vi "Main.vi"(8 "error in (no error)":errorcluster, 11 "ModuleAdmin":refnum<class "ModuleAdmin.lvclass">) -> ()   [LabVIEW 2014, in "MyPluggableModule.lvlib"]
uses:
  MyPluggableModule.lvlib
  <userlib>/NIST/ModuleAdminLib/ModuleAdmin/ModuleAdmin.lvclass
  MyPlugins/MyPluginBaseClass/MyPluginsBase.lvclass
  PublicAPI/Arguments/Requests/clStopArgument.ctl
  <userlib>/NIST/ModuleAdminLib/ModuleAdmin/ModuleAdmin.lvclass/ModuleAdmin.ctl
  <userlib>/NIST/BaseClasses/BasePlugin_class/BasePlugin.lvclass/BasePlugin.ctl
  <vilib>/Utility/error.llb/DialogType.ctl
  <userlib>/NIST/ModuleAdminLib/ModuleAdmin/Accessors/Read ShowPanel_.vi
  <userlib>/NIST/ModuleAdminLib/ModuleAdmin/Accessors/Write ShowPanel_.vi
  <userlib>/NIST/BaseClasses/BasePlugin_class/Accessors/Write PluginIniFilePath.vi
  <userlib>/NIST/BaseClasses/BasePlugin_class/Accessors/Read PluginIniFilePath.vi
  <userlib>/NIST/ModuleAdminLib/ModuleAdmin/Accessors/Read CloneRegRef.vi
  <vilib>/Utility/error.llb/Error Cluster From Error Code.vi
  <vilib>/ErrorRing/Error Ring.xnode
  <userlib>/NIST/ModuleAdminLib/CloneRegistration/CloneRegistration.lvclass
  <userlib>/NIST/BaseClasses/Object_class/BaseObject.lvclass
  <userlib>/NIST/ModuleAdminLib/ModuleAdmin.lvlib
panel:
  out "error out":errorcluster
  # "This is the template for your cloneable module.\nYou should modifiy this to perform the functionality\nthat you want it to perform"
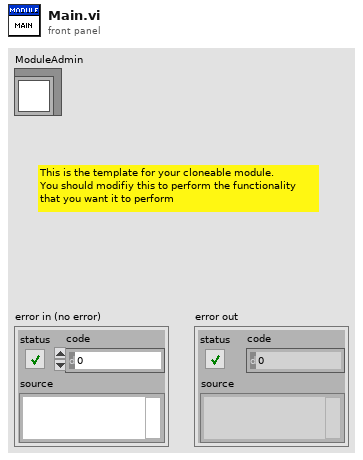
[diagram p1: front panel]
types:
  T1 = typedef "MyPluggableModule.lvlib/clRequestEvents.ctl" = cluster{"StopRequest":refnum<user-event>, "PathToINI":refnum<user-event>, " LoadPlugin":refnum<user-event>, "ShowPanel":refnum<user-event>, "PrefDlg":refnum<user-event>}
  T2 = typedef "MyPluggableModule.lvlib/clBroadcastEvents.ctl" = cluster{"DidInit":refnum<user-event>, "StatusUpdate":refnum<user-event>, "ErrorReport":refnum<user-event>, "DidStop":refnum<user-event>, "PathToINI":refnum<user-event>}
  T3 = typedef "MyPluggableModule.lvlib/clStopArgument.ctl" = cluster{"Exit via Stop Module Req?":bool, "Wait for Module to stop?":bool, "ModuleAdmin":refnum<class "ModuleAdmin.lvclass">}
  T4 = enum32{"Invalid", "Standard", "Closed", "Hidden", "Minimized", "Maximized"}
  T5 = typedef "DialogType.ctl" = u16
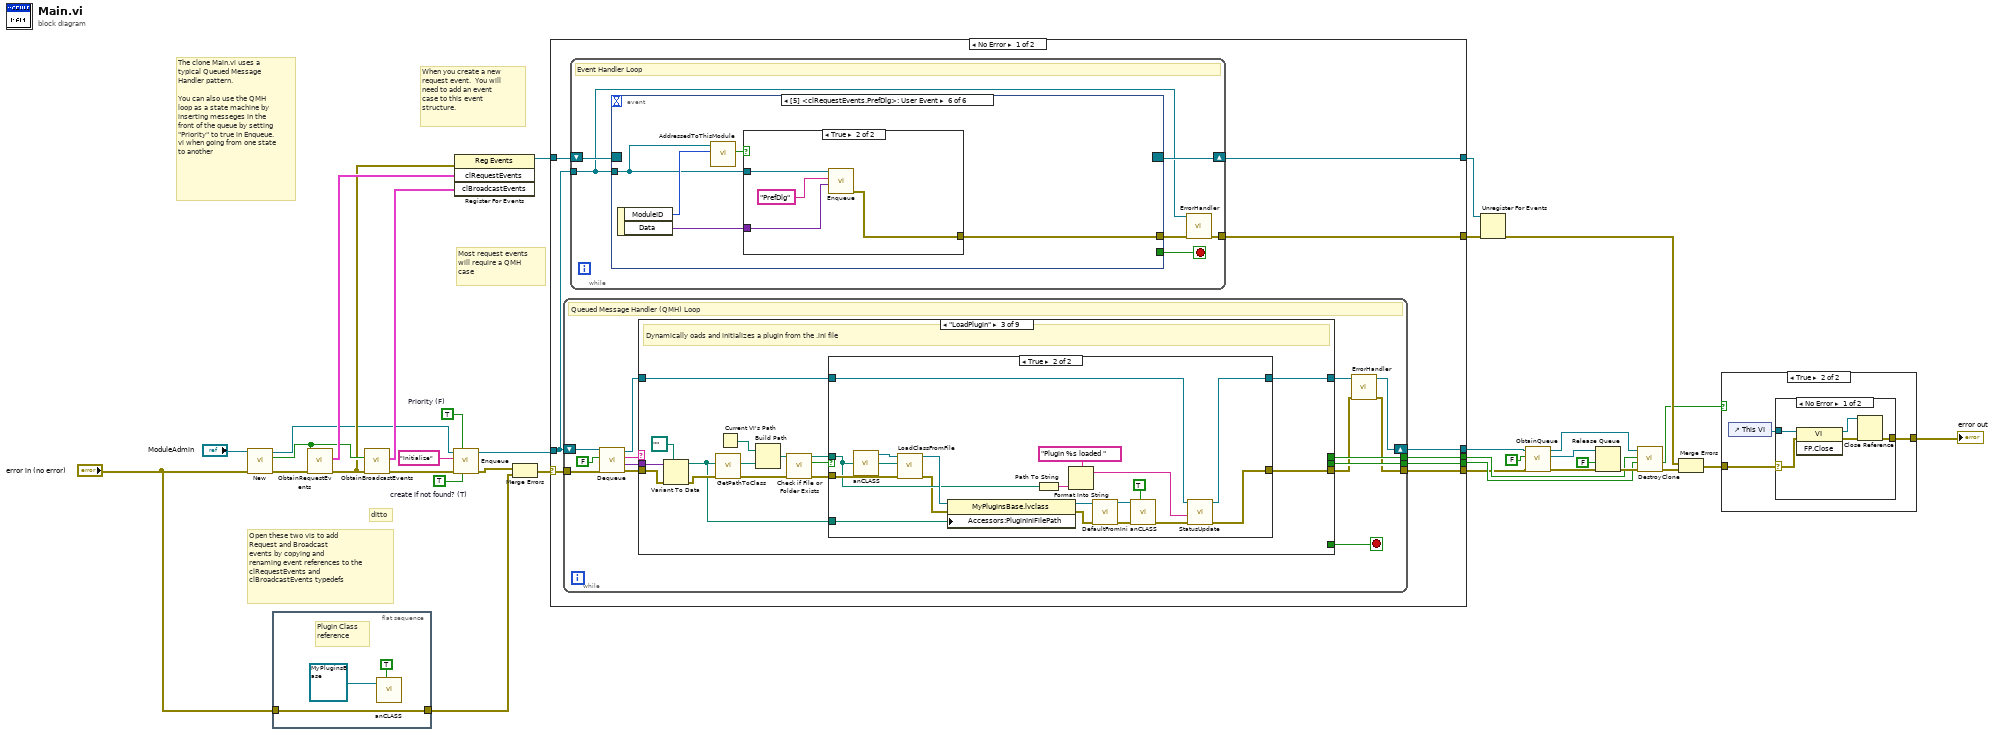
[diagram p0: block diagram]
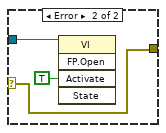
[diagram p3: hidden frame]
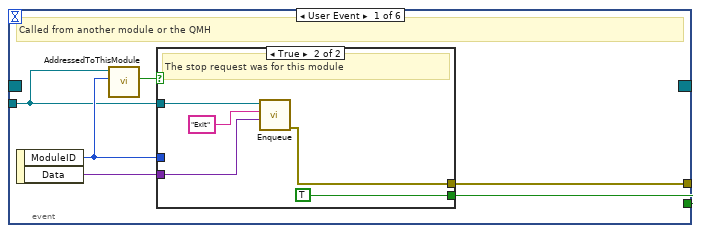
[diagram p4: hidden frame]
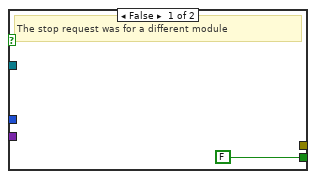
[diagram p5: hidden frame]
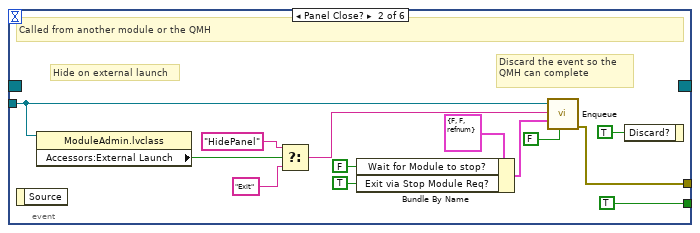
[diagram p6: hidden frame]
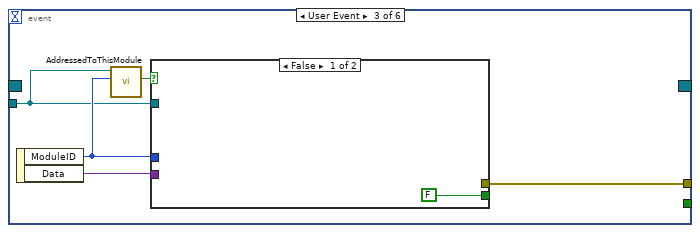
[diagram p7: hidden frame]
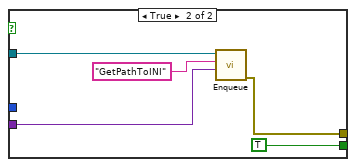
[diagram p8: hidden frame]
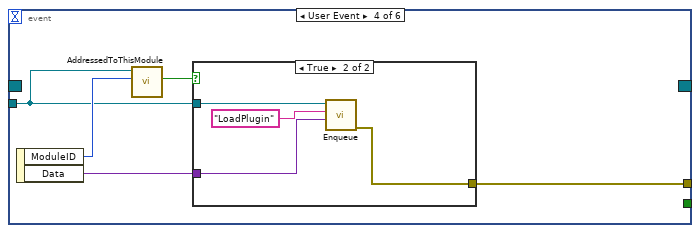
[diagram p9: hidden frame]
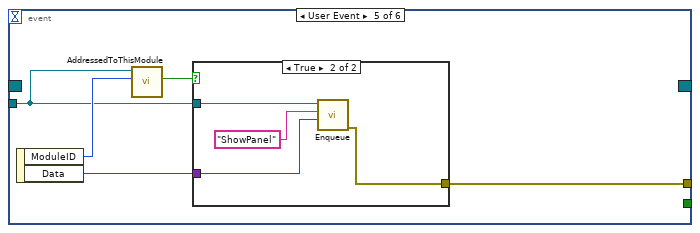
[diagram p11: hidden frame]
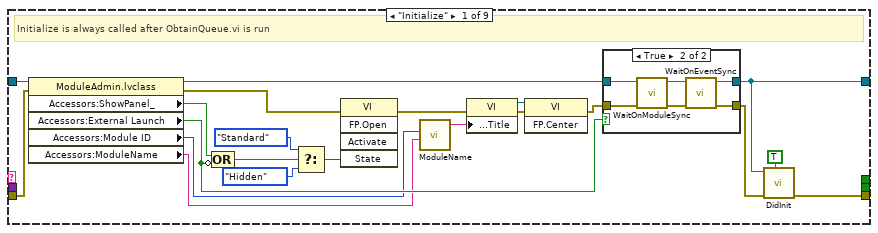
[diagram p14: hidden frame]
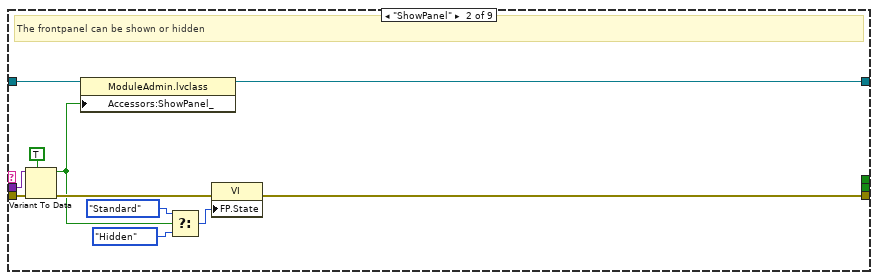
[diagram p16: hidden frame]
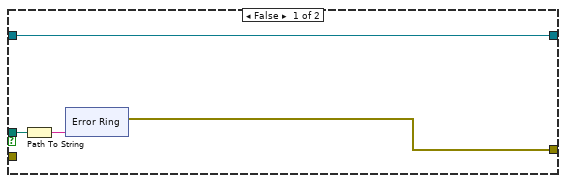
[diagram p17: hidden frame]
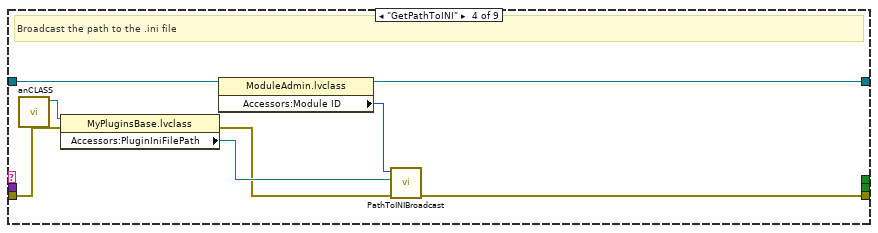
[diagram p18: hidden frame]
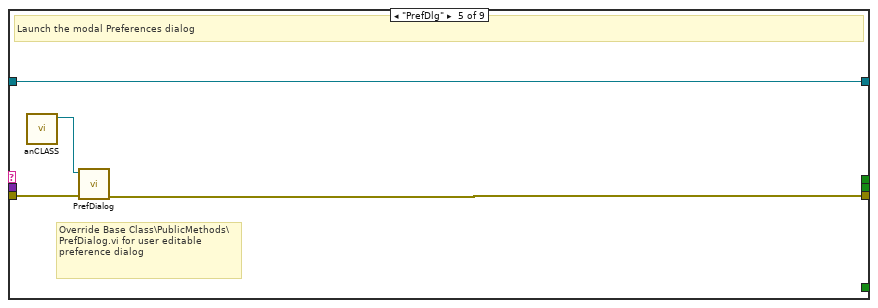
[diagram p19: hidden frame]
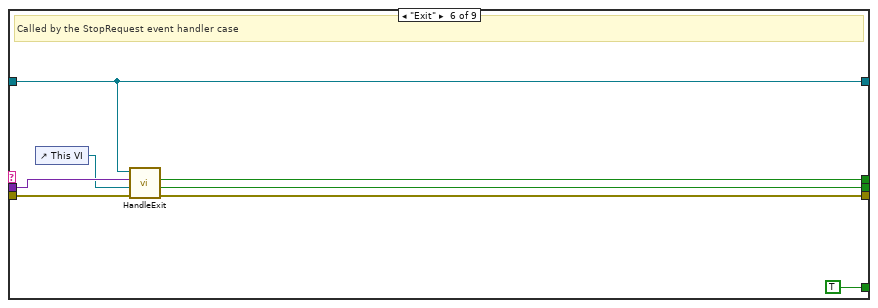
[diagram p20: hidden frame]
diagram:
  w16 = TRUE  # create if not found? (T)
  w17 = TRUE  # Priority (F)
  # "The clone Main.vi uses a typical Queued Message Handler pattern.  \n\nYou can also use the QMH loop as a state machine by inserting messeges in the front of the queue by setting \"Priority\" to true in Enqueue.vi when going from one state to another"
  # "Open these two vis to add\nRequest and Broadcast \nevents by copying and \nrenaming event references to the \nclRequestEvents and \nclBroadcastEvents typedefs"
  # "ditto"
  # "Most request events\nwill require a QMH\ncase"
  # "When you create a new request event.  You will need to add an event case to this event structure."
  n1 = call <userlib>:"New.vi"("error in (no error)"="error in (no error)", "ModuleAdmin"="ModuleAdmin") -> ("error out"=w24:errorcluster, "First?"=w32:bool, "ModuleAdmin"=w22:refnum<class "ModuleAdmin.lvclass">)  [unwired: 6 in, 1 out]
  n2 = flat-sequence {
    tunnel: "error in (no error)" -> [w35]
    tunnel: [w35] -> w12
    frame #0 {
      # "Plugin Class\nreference"
      n3 = call "anCLASS.vi"("Set? (f)"=TRUE, "MyPlugins.lvlib In"=refnum<class "MyPluginsBase.lvclass"> refnum ("MyPlugins.lvlib:MyPluginsBase.lvclass")) -> ()  [unwired: 9 in, 1 out]
    }
  }
  n4 = call "ObtainRequestEvents.vi"("error in (no error)"=w24, "CreateNew (F)"=w32) -> ("error out"=w31:errorcluster, "clRequestEvents"=w33:T1)  [unwired: 8 in]
  n5 = call "ObtainBroadcastEvents.vi"("error in (no error)"=w31, "CreateNew? (F)"=w32) -> ("error out"=w23:errorcluster, "clBroadcastEvents"=w30:T2)  [unwired: 8 in]
  n6 = call "Enqueue.vi"("create if not found? (T)"=w16, "Priority (F)"=w17, "error in (no error)"=w23, "Message"="Initialize", "ModuleAdmin"=w22) -> ("error out"=w13:errorcluster, "ModuleAdmin Out"=w21:refnum<class "ModuleAdmin.lvclass">)  [unwired: 5 in]
  n7 = register-events(error in=w31, w33, w30) -> (reference out=w29:refnum<event-registration>)  [unwired: 1 in, 1 out]
  n8 = Merge Errors(w13, w12) -> (w14:errorcluster)
  n9 = case shown="No Error" w14 {
    selector: w14 -> [w46 w277]
    tunnel: w21 -> [w39 w270]
    tunnel: [w38 w275] -> w2
    tunnel: w29 -> [w45 w271]
    tunnel: [w44 w274] -> w3
    tunnel: [w43 _] -> w6
    tunnel: [w42 _] -> w5
    tunnel: [w41 _] -> w28
    tunnel: [w40 w271] -> w27
    frame No Error {
      n10 = while {
        tunnel: w46 -> [w128]
        tunnel: [w122] -> w38
        tunnel: [w124] -> w43
        tunnel: [w123] -> w42
        shift-right: [w119] -> w44
        shift-left: w39 -> [w118]
        stop <- w129 stop-if-true
        # "Queued Message Handler (QMH) Loop"
        n11 = call "Dequeue.vi"("error in (no error)"=w128, "create if not found? (f)"=FALSE ("create if not found? (T)"), "ModuleAdmin"=w118) -> ("error out"=w127:errorcluster, "Message Data"=w125:variant, "Message"=w126:string, "ModuleAdmin Out"=w117:refnum<class "ModuleAdmin.lvclass">)  [unwired: 5 in]
        n12 = case shown="\"LoadPlugin\"" w126 {
          selector: w126 -> [_ _ _ _ _ _ _ _ w258]
          tunnel: [_ _ _ _ _ TRUE _ TRUE _] -> w129
          tunnel: w117 -> [w150 w166 w172 w218 w222 w225 w234 w251 w261]
          tunnel: [w139 w159 w173 w219 w223 w231 w235 w253 w257] -> w121
          tunnel: w127 -> [w132 w169 w182 w216 w224 w230 w243 _ _]
          tunnel: w125 -> [_ w168 w184 _ _ w229 w242 _ _]
          tunnel: [_ _ _ _ _ w227 _ _ _] -> w124
          tunnel: [_ _ _ _ _ w226 _ _ _] -> w123
          tunnel: [w133 w165 w170 w214 w222 w225 w233 w251 w255] -> w120
          frame "Initialize" {
            # "Initialize is always called after ObtainQueue.vi is run"
            n13 = property class="ModuleAdmin.lvclass"(reference=w150, error in=w132) -> (reference out=w137:refnum<class "ModuleAdmin.lvclass">, error out=w147:errorcluster, "Accessors:ShowPanel_"=w136:bool, "Accessors:External Launch"=w135:bool, "Accessors:Module ID"=w130:i32, "Accessors:ModuleName"=w131:string)
            n14 = Compound Arithmetic op=OR(w136, invert w135) -> (w134:bool)
            n15 = Select(t=T4."Standard" ("Front Panel Window:State"), s=w134, f=T4."Hidden" ("Front Panel Window:State")) -> (s? t:f=w143:T4)
            n16 = invoke class="VI" method="FP.Open"(error in=w147, "State"=w143) -> (error out=w146:errorcluster)  [unwired: 3 in, 4 out]
            n17 = call <userlib>:"ModuleName.vi"("Name"=w131, "ModuleID"=w130) -> ("ModuleName"=w142:string)  [unwired: 9 in]
            n18 = property class="VI"(error in=w146, "Front Panel.Title"=w142) -> (reference out=w149:refnum<vi>, error out=w148:errorcluster)  [unwired: 1 in]
            n19 = invoke class="VI" method="FP.Center"(reference=w149, error in=w148) -> (error out=w138:errorcluster)  [unwired: 1 in, 2 out]
            n20 = case shown="True" w135 {
              tunnel: [w151 w157] -> w140
              tunnel: [w152 w154] -> w133
              tunnel: w138 -> [w151 w156]
              tunnel: w137 -> [w152 w153]
              frame False {
              }
              frame True {
                n21 = call <userlib>:"WaitOnModuleSync.vi"("error in (no error)"=w156, "ModuleAdmin"=w153) -> ("error out"=w158:errorcluster, "ModuleAdmin"=w155:refnum<class "ModuleAdmin.lvclass">)  [unwired: 8 in]
                n22 = call <userlib>:"WaitOnEventSync.vi"("error in (no error)"=w158, "ModuleAdmin"=w155) -> ("error out"=w157:errorcluster, "ModuleAdmin"=w154:refnum<class "ModuleAdmin.lvclass">)  [unwired: 8 in]
              }
            }
            n23 = call "DidInit.vi"("Init?"=TRUE, "error in (no error)"=w140, "ModuleAdmin"=w133) -> ("error out"=w139:errorcluster)  [unwired: 8 in]
          }
          frame "ShowPanel" {
            # "The frontpanel can be shown or hidden"
            n24 = Variant To Data(error in=w169, type=TRUE, Variant=w168) -> (data=w161:bool, error out=w164:errorcluster)
            n25 = property class="ModuleAdmin.lvclass"(reference=w166, "Accessors:ShowPanel_"=w161) -> (reference out=w165:refnum<class "ModuleAdmin.lvclass">)  [unwired: 1 in, 1 out]
            n26 = Select(t=T4."Standard" ("Front Panel Window:State"), s=w161, f=T4."Hidden" ("Front Panel Window:State")) -> (s? t:f=w160:T4)
            n27 = property class="VI"(error in=w164, "FP.State"=w160) -> (error out=w159:errorcluster)  [unwired: 1 in, 1 out]
          }
          frame "LoadPlugin" {
            # "Dynamically oads and initializes a plugin from the .ini file"
            n28 = Variant To Data(error in=w182, type=path "", Variant=w184) -> (data=w171:path, error out=w181:errorcluster)
            n29 = call <userlib>:"GetPathToClass.vi"("error in (no error)"=w181, "configuration file path"=w171) -> ("error IO"=w177:errorcluster, "PathToClass"=w180:path)  [unwired: 8 in]
            n30 = Current VI's Path() -> (path=w179:path)
            n31 = Build Path(base path=w179, name or relative path=w180) -> (appended path=w178:path)
            n32 = call <vilib>:"Check if File or Folder Exists.vi"("error in (no error)"=w177, "path"=w178) -> ("error out"=w174:errorcluster, "file or folder exists?"=w176:bool, "dup path"=w175:path)  [unwired: 7 in]
            n33 = case shown="True" w176 {
              tunnel: w175 -> [w187 w206]
              tunnel: w174 -> [_ w212]
              tunnel: [w186 w208] -> w173
              tunnel: w172 -> [w185 w203]
              tunnel: w171 -> [_ w204]
              tunnel: [w185 w202] -> w170
              frame False {
                n34 = Path To String(path=w187) -> (string=w188:string)
                n35 = xnode "Error Ring"("parameter 0"=w188) -> ("error out"=w186:errorcluster)
              }
              frame True {
                n36 = call "anCLASS.vi"() -> ("MyPlugins.lvlib Out"=w198:refnum<class "MyPluginsBase.lvclass">)  [unwired: 11 in]
                n37 = call-dynamic "LoadClassFromFile.vi"("error in (no error)"=w212, "class path"=w206, "reference in"=w198) -> ("error out"=w205:errorcluster, "reference out"=w207:refnum<class "MyPluginsBase.lvclass">)  [unwired: 7 in]
                n38 = property class="MyPluginsBase.lvclass"(reference=w207, error in=w205, "Accessors:PluginIniFilePath"=w204) -> (reference out=w201:refnum<class "MyPluginsBase.lvclass">, error out=w200:errorcluster)
                n39 = Path To String(path=w206) -> (string=w210:string)
                n40 = Format Into String(format string="Plugin %s loaded ", w210) -> (resulting string=w209:string)  [unwired: 2 in, 1 out]
                n41 = call-dynamic "DefaultFromIni.vi"("error in (no error)"=w200, "MyPluginsBase in"=w201) -> ("error out"=w199:errorcluster, "MyPluginsBase out"=w197:refnum<class "MyPluginsBase.lvclass">)  [unwired: 8 in]
                n42 = call "anCLASS.vi"("Set? (f)"=TRUE, "MyPlugins.lvlib In"=w197) -> ()  [unwired: 9 in, 1 out]
                n43 = call "StatusUpdate.vi"("error in (no error)"=w199, "Status"=w209, "Module"=w203) -> ("error out"=w208:errorcluster, "Module"=w202:refnum<class "ModuleAdmin.lvclass">)  [unwired: 7 in]
              }
            }
          }
          frame "GetPathToINI" {
            # "Broadcast the path to the .ini file"
            n44 = call "anCLASS.vi"() -> ("MyPlugins.lvlib Out"=w213:refnum<class "MyPluginsBase.lvclass">)  [unwired: 11 in]
            n45 = property class="MyPluginsBase.lvclass"(reference=w213, error in=w216) -> (error out=w215:errorcluster, "Accessors:PluginIniFilePath"=w217:path)  [unwired: 1 out]
            n46 = property class="ModuleAdmin.lvclass"(reference=w218) -> (reference out=w214:refnum<class "ModuleAdmin.lvclass">, "Accessors:Module ID"=w220:i32)  [unwired: 1 in, 1 out]
            n47 = call "PathToINIBroadcast.vi"("error in (no error)"=w215, "PathToINI"=w217, "ModuleID"=w220) -> ("error out"=w219:errorcluster)  [unwired: 8 in]
          }
          frame "PrefDlg" {
            # "Override Base Class\\PublicMethods\\PrefDialog.vi for user editable preference dialog"
            # "Launch the modal Preferences dialog"
            n48 = call "anCLASS.vi"() -> ("MyPlugins.lvlib Out"=w221:refnum<class "MyPluginsBase.lvclass">)  [unwired: 11 in]
            n49 = call-dynamic "PrefDialog.vi"("error in (no error)"=w224, "MyPluginsBase in"=w221) -> ("error out"=w223:errorcluster)  [unwired: 8 in, 1 out]
          }
          frame "Exit" {
            # "Called by the StopRequest event handler case"
            n50 = control-ref of="This VI"() -> (w228:refnum<vi>)
            n51 = call "HandleExit.vi"("error in (no error)"=w230, "VI Refnum"=w228, "StopArgument"=w229, "ModuleAdmin"=w225) -> ("error out"=w231:errorcluster, "Exit via Stop Module Req?"=w226:bool, "WaitForStop?"=w227:bool)  [unwired: 5 in]
          }
          frame "Error" {
            # "Handle any errors"
            n52 = property class="ModuleAdmin.lvclass"(reference=w234) -> (reference out=w233:refnum<class "ModuleAdmin.lvclass">, "Accessors:External Launch"=w238:bool, "Accessors:Module ID"=w236:i32)  [unwired: 1 in, 1 out]
            n53 = Variant To Data(error in=w243, type=errorcluster {"status"=FALSE, "code"=0, "source"=""} ("error constant"), Variant=w242) -> (data=w237:errorcluster, error out=w240:errorcluster)
            n54 = call "ReportError.vi"("error in (no error)"=w240, "ErrorReported"=w237, "ModuleID"=w236) -> ("error out"=w239:errorcluster)  [unwired: 8 in]
            n55 = case shown="False" w238 {
              tunnel: w239 -> [w247 w248]
              tunnel: w237 -> [w246 _]
              tunnel: [w245 w248] -> w235
              tunnel: w234 -> [w244 _]
              frame False {
                # "Todo:  Add an event to ask the user\nIf the module should stop or continue"
                # "Stand alone: now, force an exit"
                n56 = call <vilib>:"Simple Error Handler.vi"("error in (no error)"=w246) -> ()  [unwired: 4 in, 5 out]
                n57 = call "StopRequest.vi"("error in (no error)"=w247, "ModuleAdmin"=w244) -> ("error out"=w245:errorcluster)  [unwired: 8 in, 1 out]
              }
              frame True {
                # "Externally launched modules only broadcast the error msg"
              }
            }
          }
          frame "QueueError" {
            n58 = call "StatusUpdate.vi"("Status"=" Queue Error" ("format string"), "Module"=w251) -> ("error out"=w254:errorcluster, "Module"=w252:refnum<class "ModuleAdmin.lvclass">)  [unwired: 8 in]
            n59 = call "StopRequest.vi"("error in (no error)"=w254, "ModuleAdmin"=w252) -> ("error out"=w253:errorcluster)  [unwired: 8 in, 1 out]
          }
          frame Default {
            # "Called only if a message was queued and no QMH case was created"
            n60 = property class="ModuleAdmin.lvclass"(reference=w261) -> (reference out=w255:refnum<class "ModuleAdmin.lvclass">, "Accessors:Module ID"=w260:i32, "Accessors:ModuleName"=w256:string)  [unwired: 1 in, 1 out]
            n61 = call <userlib>:"ModuleName.vi"("Name"=w256, "ModuleID"=w260) -> ("ModuleName"=w259:string)  [unwired: 9 in]
            n62 = xnode "Error Ring"("parameter 0"=w258, "parameter 1"=w259) -> ("error out"=w257:errorcluster)
          }
        }
        n63 = call "ErrorHandler.vi"("error in (no error)"=w121, "ModuleAdmin"=w120) -> ("error out"=w122:errorcluster, "ModuleAdmin Out"=w119:refnum<class "ModuleAdmin.lvclass">)  [unwired: 8 in]
      }
      n64 = while {
        tunnel: w39 -> [w47]
        shift-right: [w50] -> w40
        shift-left: w45 -> [w51]
        tunnel: [w48] -> w41
        stop <- w52 stop-if-true
        # "Event Handler Loop"
        n65 = event shown="[5] <clRequestEvents.PrefDlg>: User Event" {
          selector: w51 -> [_ _ _ _ _ _]
          dyn-events: [_ _ _ _ _ _] -> w50
          timeout: _ -> [_ _ _ _ _ _]
          tunnel: w47 -> [w53 w66 w78 w89 w98 w107]
          tunnel: [w56 TRUE _ _ _ _] -> w52
          tunnel: [w55 w76 w79 w91 w100 w109] -> w49
          event User Event {
            # "Called from another module or the QMH"
            n66 = event-data() -> ("ModuleID"=w57:i32, "Data"=w54:variant)  [unwired: 1 in]
            n67 = call <userlib>:"AddressedToThisModule.vi"("ModuleID"=w57, "ModuleAdmin"=w53) -> ("AddressedToThisInstance?"=w58:bool)  [unwired: 8 in, 1 out]
            n68 = case shown="True" w58 {
              tunnel: w57 -> [_ _]
              tunnel: w53 -> [_ w64]
              tunnel: [FALSE TRUE] -> w56
              tunnel: [_ w62] -> w55
              tunnel: w54 -> [_ w60]
              frame False {
                # "The stop request was for a different module"
              }
              frame True {
                # "The stop request was for this module"
                n69 = call "Enqueue.vi"("Message Data"=w60, "Message"="Exit", "ModuleAdmin"=w64) -> ("error out"=w62:errorcluster)  [unwired: 7 in, 1 out]
              }
            }
          }
          event Panel Close? {
            # "Hide on external launch"
            # "Discard the event so the QMH can complete"
            # "Called from another module or the QMH"
            n70 = event-data() -> ()  [unwired: 1 in, 1 out]
            n71 = property class="ModuleAdmin.lvclass"(reference=w66) -> ("Accessors:External Launch"=w68:bool)  [unwired: 1 in, 2 out]
            n72 = Select(t="HidePanel", s=w68, f="Exit" ("Message")) -> (s? t:f=w70:string)
            n73 = Bundle By Name(cluster=T3 {"Exit via Stop Module Req?"=FALSE, "Wait for Module to stop?"=FALSE, "ModuleAdmin"=refnum} ("Stop Argument"), "Wait for Module to stop?"=FALSE, "Exit via Stop Module Req?"=TRUE) -> (w73:T3)
            n74 = call "Enqueue.vi"("create if not found? (T)"=FALSE, "Message Data"=w73, "Message"=w70, "ModuleAdmin"=w66) -> ("error out"=w76:errorcluster)  [unwired: 6 in, 1 out]
            n75 = event-data("Discard?"=TRUE) -> ()  [unwired: 1 in, 1 out]
          }
          event User Event {
            n76 = event-data() -> ("ModuleID"=w80:i32, "Data"=w81:variant)  [unwired: 1 in]
            n77 = call <userlib>:"AddressedToThisModule.vi"("ModuleID"=w80, "ModuleAdmin"=w78) -> ("AddressedToThisInstance?"=w82:bool)  [unwired: 8 in, 1 out]
            n78 = case shown="False" w82 {
              tunnel: w80 -> [_ _]
              tunnel: w78 -> [_ w88]
              tunnel: [FALSE TRUE] -> _
              tunnel: [_ w86] -> w79
              tunnel: w81 -> [_ w84]
              frame False {
                # "The stop request was for a different module"
              }
              frame True {
                # "The stop request was for this module"
                n79 = call "Enqueue.vi"("Message Data"=w84, "Message"="GetPathToINI", "ModuleAdmin"=w88) -> ("error out"=w86:errorcluster)  [unwired: 7 in, 1 out]
              }
            }
          }
          event User Event {
            n80 = event-data() -> ("ModuleID"=w93:i32, "Data"=w90:variant)  [unwired: 1 in]
            n81 = call <userlib>:"AddressedToThisModule.vi"("ModuleID"=w93, "ModuleAdmin"=w89) -> ("AddressedToThisInstance?"=w92:bool)  [unwired: 8 in, 1 out]
            n82 = case shown="True" w92 {
              tunnel: [_ w94] -> w91
              tunnel: w89 -> [_ w97]
              tunnel: w90 -> [_ w95]
              frame False {
              }
              frame True {
                n83 = call "Enqueue.vi"("Message Data"=w95, "Message"="LoadPlugin", "ModuleAdmin"=w97) -> ("error out"=w94:errorcluster)  [unwired: 7 in, 1 out]
              }
            }
          }
          event User Event {
            n84 = event-data() -> ("ModuleID"=w102:i32, "Data"=w99:variant)  [unwired: 1 in]
            n85 = call <userlib>:"AddressedToThisModule.vi"("ModuleID"=w102, "ModuleAdmin"=w98) -> ("AddressedToThisInstance?"=w101:bool)  [unwired: 8 in, 1 out]
            n86 = case shown="True" w101 {
              tunnel: [_ w103] -> w100
              tunnel: w98 -> [_ w106]
              tunnel: w99 -> [_ w104]
              frame False {
              }
              frame True {
                n87 = call "Enqueue.vi"("Message Data"=w104, "Message"="ShowPanel", "ModuleAdmin"=w106) -> ("error out"=w103:errorcluster)  [unwired: 7 in, 1 out]
              }
            }
          }
          event User Event {
            n88 = event-data() -> ("ModuleID"=w111:i32, "Data"=w108:variant)  [unwired: 1 in]
            n89 = call <userlib>:"AddressedToThisModule.vi"("ModuleID"=w111, "ModuleAdmin"=w107) -> ("AddressedToThisInstance?"=w110:bool)  [unwired: 8 in, 1 out]
            n90 = case shown="True" w110 {
              tunnel: [_ w112] -> w109
              tunnel: w107 -> [_ w115]
              tunnel: w108 -> [_ w113]
              frame False {
              }
              frame True {
                n91 = call "Enqueue.vi"("Message Data"=w113, "Message"="PrefDlg", "ModuleAdmin"=w115) -> ("error out"=w112:errorcluster)  [unwired: 7 in, 1 out]
              }
            }
          }
        }
        n92 = call "ErrorHandler.vi"("error in (no error)"=w49, "ModuleAdmin"=w47) -> ("error out"=w48:errorcluster)  [unwired: 8 in, 1 out]
      }
    }
    frame Error {
      n93 = property class="ModuleAdmin.lvclass"(reference=w270) -> (reference out=w274:refnum<class "ModuleAdmin.lvclass">, "Accessors:CloneRegRef"=w273:refnum<data-value>, "Accessors:Module ID"=w272:i32)  [unwired: 1 in, 1 out]
      n94 = call <userlib>:"Remove.vi"("Module ID"=w272, "CloneRegRef"=w273) -> ("error out"=w276:errorcluster)  [unwired: 7 in, 2 out]
      n95 = flat-sequence {
        tunnel: w277 -> [w280]
        tunnel: w276 -> [_]
        tunnel: [w278] -> w275
        frame #0 {
          w279 = T5 2 items=["no dialog", "OK message", "continue or stop message", "OK message + warnings", "continue/stop + warnings"] ("type of dialog (OK msg:1)")
          n96 = call <vilib>:"Simple Error Handler.vi"("type of dialog (OK msg:1)"=w279, "error in (no error)"=w280) -> ("error out"=w278:errorcluster)  [unwired: 3 in, 4 out]
        }
      }
    }
  }
  n97 = Unregister For Events(event registration refnum=w27, error in=w28) -> (error out=w26:errorcluster)
  n98 = call "ObtainQueue.vi"("error in (no error)"=w2, "create if not found? (f)"=FALSE ("create if not found? (T)"), "ModuleAdmin"=w3) -> ("error out"=w11:errorcluster, "queue out"=w19:refnum<queue>, "ModuleAdmin Out"=w7:refnum<class "ModuleAdmin.lvclass">)  [unwired: 6 in]
  n99 = Release Queue(queue=w19, force destroy? (F)=FALSE, error in (no error)=w11) -> (error out=w9:errorcluster)  [unwired: 2 out]
  n100 = call "DestroyClone.vi"("error in (no error)"=w9, "Exit via Stop Module Req?"=w5, "Wait for Module to stop?"=w6, "ModuleAdmin"=w7) -> ("error out"=w8:errorcluster, "External Launch"=w4:bool)  [unwired: 5 in, 1 out]
  n101 = Merge Errors(w26, w8) -> (w10:errorcluster)
  n102 = case shown="True" w4 {
    tunnel: w10 -> [w281 w284]
    tunnel: [w281 w282] -> w1
    frame False {
    }
    frame True {
      n103 = control-ref of="This VI"() -> (w283:refnum<vi>)
      n104 = case shown="No Error" w284 {
        selector: w284 -> [w288 w290]
        tunnel: w283 -> [w289 w291]
        tunnel: [w285 w290] -> w282
        frame No Error {
          n105 = invoke class="VI" method="FP.Close"(reference=w289, error in=w288) -> (reference out=w286:refnum<vi>, error out=w287:errorcluster)  [unwired: 1 in, 1 out]
          n106 = Close Reference(reference=w286, error in (no error)=w287) -> (error out=w285:errorcluster)
        }
        frame Error {
          n107 = invoke class="VI" method="FP.Open"(reference=w291, "Activate"=TRUE ("Activate?")) -> ()  [unwired: 3 in, 5 out]
        }
      }
    }
  }
  "error out" <- w1
